vi "View Song Library Request by Artist.vi"(8 "error in (no error)":errorcluster, 10 "Artist":string, 11 "MusicManagerActor in":refnum<class "MusicManagerActor.lvclass">) -> (0 "error out":errorcluster, 3 "MusicManagerActor out":refnum<class "MusicManagerActor.lvclass">)   [LabVIEW 2015, in "MusicManagerActor.lvlib" / "MusicManagerActor.lvclass"]
uses:
  MusicManagerActor.lvclass
  MusicManagerActor.lvclass/MusicManagerActor.ctl
  SongBrowserActor/SongBrowserActor Messages/Display Song Library Msg/Display Song Library Msg.lvclass
  file/MusicElement/MusicElementLibrary/MusicLibrary/MusicLibrary.lvclass
  SongQueueActor/SongQueueActor Messages/Set Visibility Of Queue List Msg/Set Visibility Of Queue List Msg.lvclass
  file/MusicElement/MusicElementLibrary/SongLibrary/SongLibrary.lvclass
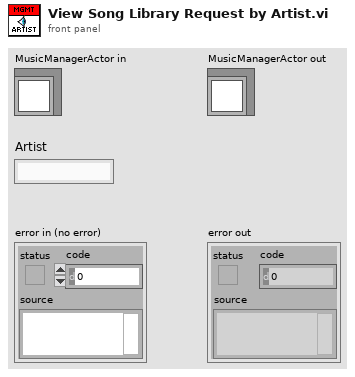
[diagram p1: front panel]
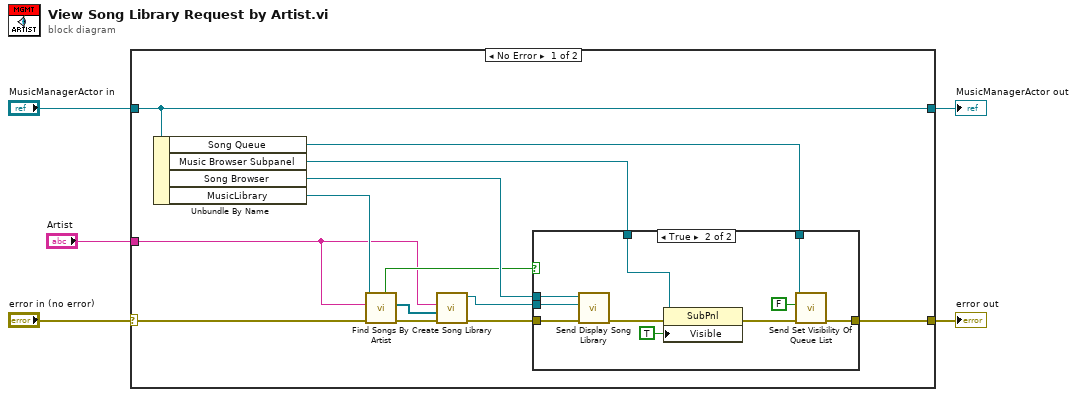
[diagram p0: block diagram]
diagram:
  n1 = case shown="No Error" "error in (no error)" {
    selector: "error in (no error)" -> [w14 w31]
    tunnel: [w17 w31] -> w4
    tunnel: [w18 w30] -> w2
    tunnel: "MusicManagerActor in" -> [w18 w30]
    tunnel: "Artist" -> [w9 _]
    frame No Error {
      n2 = Unbundle By Name(w18) -> ("Song Queue"=w11:refnum<class "Message Enqueuer.lvclass">, "Music Browser Subpanel"=w16:refnum<vi>, "Song Browser"=w15:refnum<class "Message Enqueuer.lvclass">, "MusicLibrary"=w13:refnum<class "MusicLibrary.lvclass">)
      n3 = call "Find Songs By Artist.vi"("error in (no error)"=w14, "Artist"=w9, "MusicLibrary in"=w13) -> ("error out"=w10:errorcluster, "Songs"=w8:refnum<class "Song.lvclass">[], "Found?"=w12:bool)  [unwired: 5 in, 1 out]
      n4 = call "Create Song Library.vi"("error in (no error)"=w10, "Songs"=w8, "Name"=w9) -> ("error out"=w7:errorcluster, "SongLibrary out"=w6:refnum<class "SongLibrary.lvclass">)  [unwired: 7 in]
      n5 = case shown="True" w12 {
        tunnel: [w19 w21] -> w17
        tunnel: w16 -> [_ w29]
        tunnel: w15 -> [_ w26]
        tunnel: w6 -> [_ w25]
        tunnel: w7 -> [w19 w24]
        tunnel: w11 -> [_ w20]
        frame False {
        }
        frame True {
          n6 = call "Send Display Song Library.vi"("error in (no error)"=w24, "Song Library"=w25, "Message Enqueuer in"=w26) -> ("error out"=w27:errorcluster)  [unwired: 7 in, 1 out]
          n7 = property class="SubPnl"(reference=w29, error in=w27, "Visible"=TRUE) -> (error out=w22:errorcluster)  [unwired: 1 out]
          n8 = call "Send Set Visibility Of Queue List.vi"("error in (no error)"=w22, "Visible"=FALSE, "Message Enqueuer in"=w20) -> ("error out"=w21:errorcluster)  [unwired: 7 in, 1 out]
        }
      }
    }
    frame Error {
    }
  }
  "error out" <- w4
  "MusicManagerActor out" <- w2
